vi "v2 ap get num accesspoints on host.vi"(11 "dest":u32) -> (2 "function return":i32, 3 "dest out":u32)   [LabVIEW 2019, in "apdm.lvlib"]
doc: "APDM_EXPORT int apdm_v2_ap_get_num_accesspoints_on_host(uint32_t *dest);"
uses:
  apdm.lvlib
  Lee Lab/CP FES Walking 2018/Code/Working/LabVIEW/apdm.dll
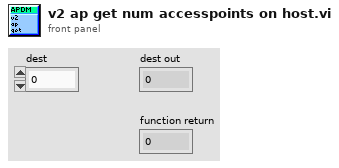
[diagram p1: front panel]
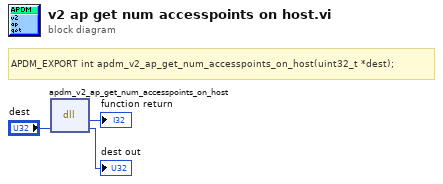
[diagram p0: block diagram]
diagram:
  # "APDM_EXPORT int apdm_v2_ap_get_num_accesspoints_on_host(uint32_t *dest);"
  n1 = dll-call lib="C:/Users/jfalesi/Dropbox/Lee Lab/CP FES Walking 2018/Code/Working/LabVIEW/apdm.*" fn="apdm_v2_ap_get_num_accesspoints_on_host"("dest"="dest") -> (→"function return":i32, "dest"=→"dest out":u32)  [unwired: 3 in, 2 out]
